vi "tagDB_value.vi"   [LabVIEW 2014, in "TagDB(dev).lvlib"]
doc: "[Covers: REQ_API_Value]\n[Covers: REQ_API_Value_REGEXP]"
uses:
  TagDB(dev).lvlib
  _XNode/tagDB_value.xnode/tagDB_value.xnode
  tagDB_Def.ctl
  _Support/Access/_variant.vi
  _Support/Error/_[error50002]Invalid DataType.vi
  _Support/Properties/tagDB dbChanged.vi
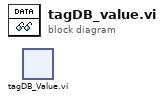
[diagram p0: block diagram]
diagram:
  n1 = xnode "tagDB_Value.vi"() -> ()  [unwired: 5 in, 3 out]
